vi "Check Cell Value is Navigatable.vi"(11 "Value":dbl) -> (3 "Invalid Cell?":bool)   [LabVIEW 2019, in "Grassfire Algorithm.lvclass"]
uses:
  Grassfire Algorithm.lvclass
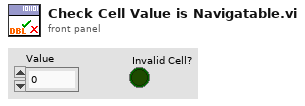
[diagram p1: front panel]
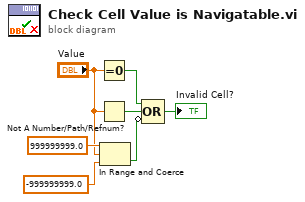
[diagram p0: block diagram]
diagram:
  n1 = Equal To 0?(x="Value") -> (x = 0?=w2:bool)
  n2 = Not A Number/Path/Refnum?(number/path/refnum="Value") -> (NaN/Path/Refnum?=w1:bool)
  n3 = In Range and Coerce(upper limit=999999999.0, x="Value", lower limit=-999999999.0) -> (In Range?=w5:bool)  [unwired: 1 out]
  n4 = Compound Arithmetic op=OR(w2, w1, invert w5) -> (→"Invalid Cell?":bool)
